vi "Get File Name.vi"(8 "Error In":errorcluster, 11 "Jig name (or acronym)":string) -> (0 "Error Out":errorcluster, 2 "Current Time Stamp (now timestamp)":timestamp, 3 "The file name of the Error Log":string)   [LabVIEW 2023, in "Error Manager.lvlib" / "ErrorLog.lvlib"]
uses:
  ErrorLog.lvlib
panel:
  # "Input\nInputs to the VI"
  # "Development\nControls or indicators that are useful for development or testing, but which are not outputs of the VI."
  # "Output\nOutputs of the VI"
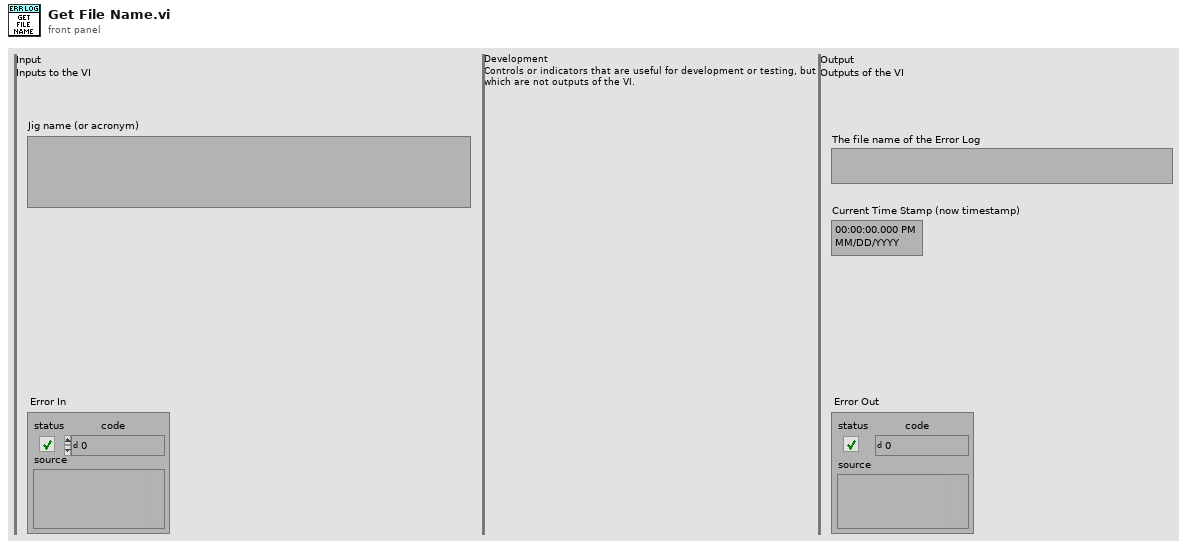
[diagram p1: front panel]
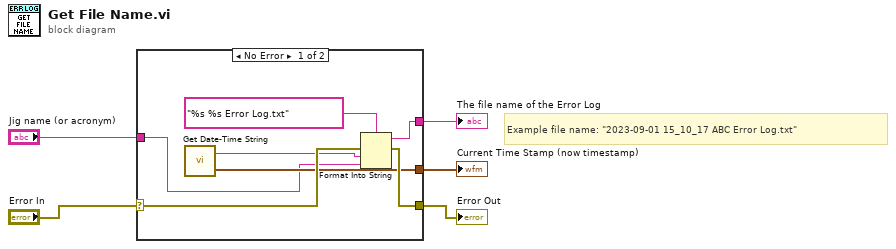
[diagram p0: block diagram]
diagram:
  # "Example file name: \"2023-09-01 15_10_17 ABC Error Log.txt\""
  n1 = case shown="No Error" "Error In" {
    selector: "Error In" -> [w10 w13]
    tunnel: [w9 w13] -> w4
    tunnel: [w11 _] -> w3
    tunnel: [w7 _] -> w2
    tunnel: "Jig name (or acronym)" -> [w6 _]
    frame No Error {
      n2 = call "Get Date-Time String.vi"() -> ("Current Time Stamp (now timestamp)"=w7:timestamp, "Date-Time String"=w8:string)  [unwired: 2 in]
      n3 = Format Into String(format string="%s %s Error Log.txt" ("time format string (%c)"), error in=w10, w8, w6) -> (resulting string=w11:string, error out=w9:errorcluster)  [unwired: 1 in]
    }
    frame Error {
    }
  }
  "Error Out" <- w4
  "The file name of the Error Log" <- w3
  "Current Time Stamp (now timestamp)" <- w2
